vi "Balloon.vi"(1 "One more?":bool, 2 "Latitude":dbl format="%#.6g", 3 "Character":string, 4 "Color":string(combo), 5 "Size":string(combo), 6 "Longitude":dbl format="%#.6g") -> (0 "Balloon":string)   [LabVIEW 2019]
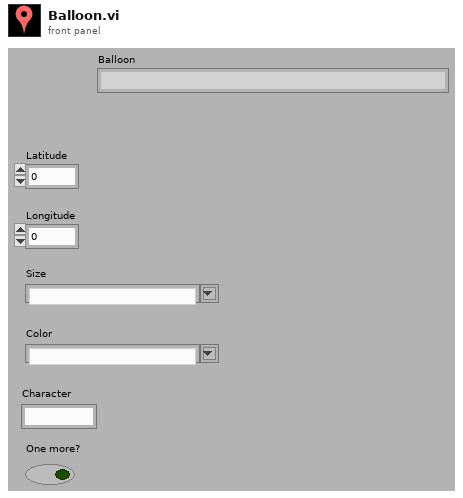
[diagram p1: front panel]
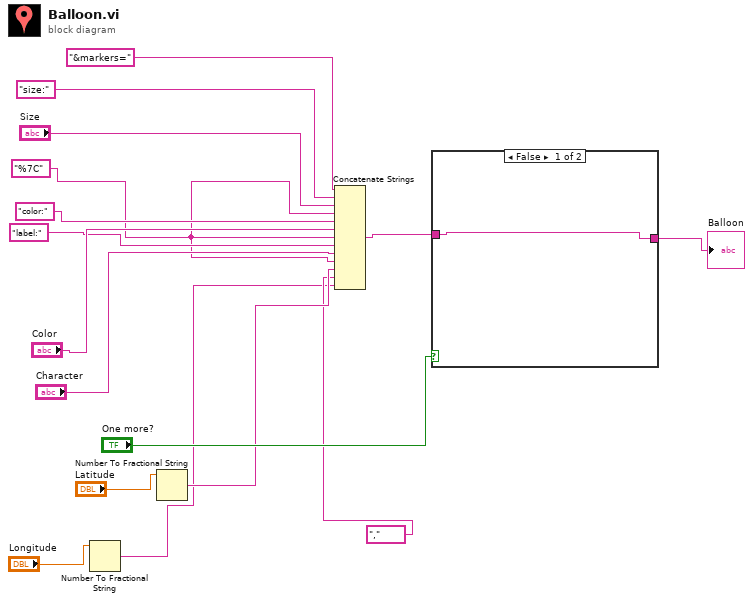
[diagram p0: block diagram]
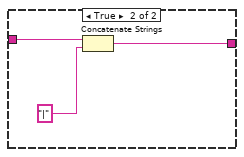
[diagram p2: hidden frame]
diagram:
  w4 = "%7C"
  n1 = Number To Fractional String(number="Longitude") -> (F-format string=w1:string)  [unwired: 3 in]
  n2 = Number To Fractional String(number="Latitude") -> (F-format string=w3:string)  [unwired: 3 in]
  n3 = Concatenate Strings("&markers=", "size:", "Size", w4, "color:", "Color", w4, "label:", "Character", w4, w3, ",", w1) -> (w12:string)
  n4 = case shown="False" "One more?" {
    tunnel: w12 -> [w17 w20]
    tunnel: [w17 w18] -> w11
    frame False {
    }
    frame True {
      n5 = Concatenate Strings(w20, "|") -> (w18:string)
    }
  }
  "Balloon" <- w11
